vi "Panther Dashboard for DQMH.vi"(8 "error in":errorcluster) -> (0 "error out":errorcluster)   [LabVIEW 2019]
doc: "Start Panther Dashboard for DQMH\n\nScan the project caller for DQMH Modules\nShow the front panel"
uses:
  Panther Dashboard.lvlib
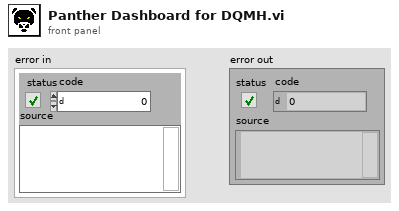
[diagram p1: front panel]
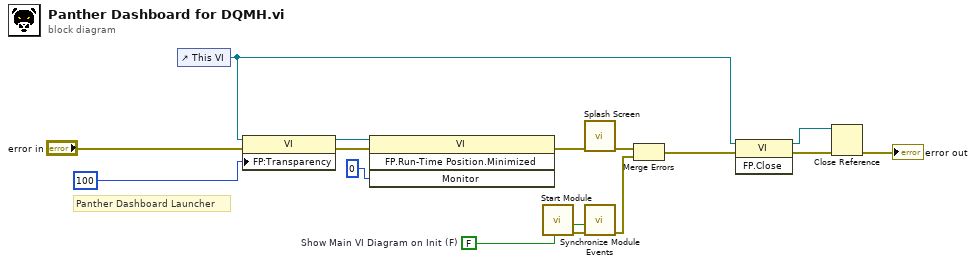
[diagram p0: block diagram]
diagram:
  w7 = FALSE  # Show Main VI Diagram on Init (F)
  # "Panther Dashboard Launcher"
  n1 = control-ref of="This VI"() -> (w3:refnum<vi>)
  n2 = property class="VI"(reference=w3, error in="error in", "FP:Transparency"=u8 100 ("Front Panel Window:Transparency")) -> (reference out=w4:refnum<vi>, error out=w13:errorcluster)
  n3 = invoke class="VI" method="FP.Run-Time Position.Minimized"(reference=w4, error in=w13, "Monitor"=i16 0) -> (error out=w14:errorcluster)  [unwired: 1 in, 3 out]
  n4 = call "Start Module.vi"("Show Main VI Diagram on Init (F)"=w7) -> ("error out"=w16:errorcluster, "Wait for Event Sync?"=w8:bool)  [unwired: 7 in, 2 out]
  n5 = call "Splash Screen.vi"("error in"=w14) -> ("error out"=w12:errorcluster)  [unwired: 10 in]
  n6 = call "Synchronize Module Events.vi"("error in"=w16, "Wait for Event Sync?"=w8) -> ("error out"=w11:errorcluster)  [unwired: 9 in]
  n7 = Merge Errors(w12, w11) -> (w9:errorcluster)
  n8 = invoke class="VI" method="FP.Close"(reference=w3, error in=w9) -> (reference out=w1:refnum<vi>, error out=w15:errorcluster)  [unwired: 1 in, 1 out]
  n9 = Close Reference(reference=w1, error in (no error)=w15) -> (error out=→"error out":errorcluster)
